vi "Configure Autotune.vi"(7 "Unit Address (1)":u8=1, 8 "error in (no error)":errorcluster, 10 "Autotune  (False: Disable)":bool, 11 "VISA resource name":refnum<visa-resource-name>) -> (0 "error out":errorcluster, 3 "VISA resource name out":refnum<visa-resource-name>)   [LabVIEW 2014, in "Eurotherm 35xx Series.lvlib"]
doc: "This VI enabled or disabled autotune. \n\nWarning: This VI is possible use only if Channel 1 Control Type value or Channel 2 Control Type value is set to \"PID\" or \"VPU\", or \"VPB\".\n\nDescription:\n\nIn tuning you match the characteristics of the controller to that of the process being controlled in order to obtain good control.\n\nGood control means:\n\nStable ‘straight-line’ control of the process at setpoint without fluctuation. \nAcceptable overshoot or undershoot of the process setpoint. \nQuick response to deviations from the setpoint caused by external disturbances, thereby restoring the process rapidly to the setpoint value. \nThe standard initial method of tuning a process loop is to use the advanced tuning algorithms inbuilt in today’s controllers, to automatically test the loop and implement the optimum PID control parameters.\n\nCare should be taken to ensure that the oscillations of the Process Value will not damage the process being tuned. It is recommended to set the Setpoint for tuning purposes below the normal running Setpoint value.\n\nThe ‘one-shot’ tuner works by switching the output on and off to induce an oscillation in the measured value. From the amplitude and period of the oscillation, it calculates the tuning parameter values.\n\nIf the process cannot tolerate full heating or cooling being applied during tuning, then the level of heating or cooling can be restricted by setting the heating and cooling power limits. However, the measured value must oscillate to some degree for the tuner to be able to calculate values.\n\nA One-shot Tune can be performed at any time, but normally it is performed only once during the initial commissioning of the process. However, if the process under control subsequently becomes unstable (because its characteristics have changed), you can re-tune again for the new conditions.\n\nIt is best to start tuning with the process at ambient temperature. This allows the tuner to calculate more accurately the low cutback and high cutback values which restrict the amount of overshoot, or undershoot."
uses:
  <instrlib>/Eurotherm 35xx Series/Eurotherm 35xx Series.lvlib
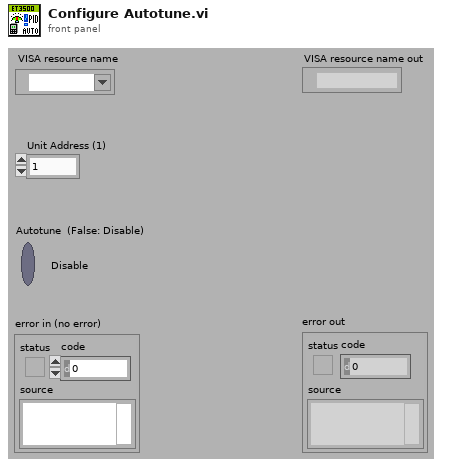
[diagram p1: front panel]
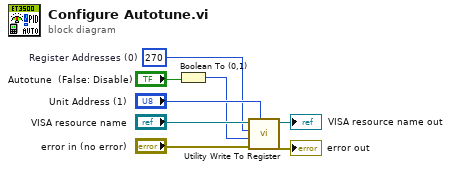
[diagram p0: block diagram]
diagram:
  w3 = 270  # Register Addresses (0)
  n1 = Boolean To (0,1)(Boolean="Autotune  (False: Disable)") -> (0, 1=w1:i16)
  n2 = call <instrlib>:"Utility Write To Register.vi"("Unit Address (1)"="Unit Address (1)", "error in (no error)"="error in (no error)", "Data (0)"=w1, "Register Address (0)"=w3, "VISA resource name"="VISA resource name") -> ("error out"=→"error out":errorcluster, "VISA resource name out"=→"VISA resource name out":refnum<visa-resource-name>)  [unwired: 5 in]
